vi "Hatch Control.vi"(10 "Driver Right Bumper":bool, 11 "Driver Left Bumper":bool) -> (3 "Hatch Intake Floor":dbl)   [LabVIEW 2018]
uses:
  <vilib>/Rock Robotics/Network Tables/NT Read Boolean.vi
  Infrastructure/Constants.vi
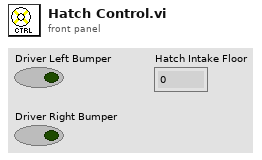
[diagram p1: front panel]
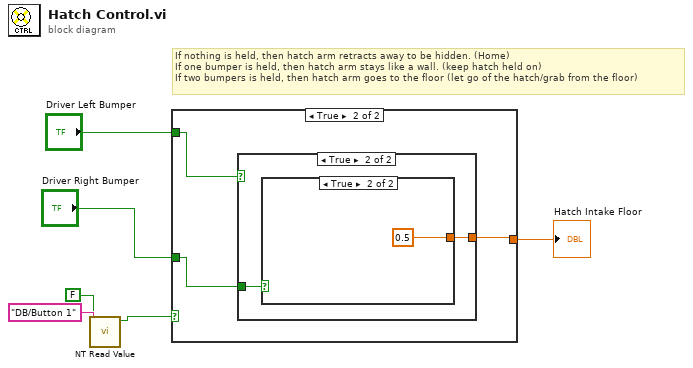
[diagram p0: block diagram]
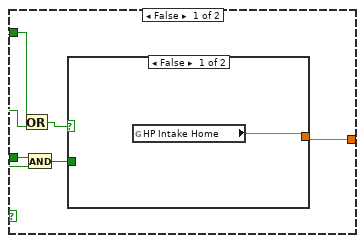
[diagram p2: hidden frame]
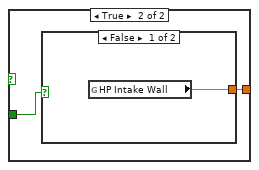
[diagram p3: hidden frame]
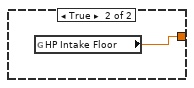
[diagram p4: hidden frame]
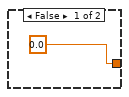
[diagram p5: hidden frame]
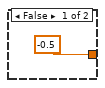
[diagram p6: hidden frame]
diagram:
  # "If nothing is held, then hatch arm retracts away to be hidden. (Home)\nIf one bumper is held, then hatch arm stays like a wall. (keep hatch held on)\nIf two bumpers is held, then hatch arm goes to the floor (let go of the hatch/grab from the floor)"
  n1 = call-poly <vilib>:"NT Read Value.vi"("Default Value"=FALSE, "Name"="DB/Button 1") -> ("Boolean"=w3:bool)  [unwired: 8 in, 1 out]
  n2 = case shown="True" w3 {
    tunnel: "Driver Right Bumper" -> [w11 w18]
    tunnel: "Driver Left Bumper" -> [w10 w19]
    tunnel: [w9 w17] -> w4
    frame False {
      n3 = Or(x=w10, y=w11) -> (x .or. y?=w7:bool)
      n4 = And(x=w11, y=w10) -> (x .and. y?=w8:bool)
      n5 = case shown="False" w7 {
        tunnel: w8 -> [_ w14]
        tunnel: [w12 w13] -> w9
        frame False {
          n6 = global read "Constants.vi" "HP Intake Home"() -> (w12:dbl)
        }
        frame True {
          n7 = case shown="False" w14 {
            tunnel: [w15 w16] -> w13
            frame False {
              n8 = global read "Constants.vi" "HP Intake Wall"() -> (w15:dbl)
            }
            frame True {
              n9 = global read "Constants.vi" "HP Intake Floor"() -> (w16:dbl)
            }
          }
        }
      }
    }
    frame True {
      n10 = case shown="True" w19 {
        tunnel: w18 -> [_ w22]
        tunnel: [0.0 w21] -> w17
        frame False {
        }
        frame True {
          n11 = case shown="True" w22 {
            tunnel: [-0.5 0.5] -> w21
            frame False {
            }
            frame True {
            }
          }
        }
      }
    }
  }
  "Hatch Intake Floor" <- w4
